vi "CRYGet Loose Curve array.vi"(8 "Unit Info In":T6={"Y unit In"="dB", "dB ref In"=1.0, "Y unit Out"="dB", "dB ref Out"=1.0, "Y unit Curve"="dB", "dB ref Curve"=1.0, "Y data  Curve"=0, "Y data Time"=0}, 9 "Loose Particle Waveform":bool, 11 "Additive Info":T2) -> (0 "Value Display Array":T4(array[cluster]), 1 "Value Unit Info Out":T5(array[cluster]), 2 "WMF Display Array":T4(array[cluster]), 3 "WFM Unit Info Out":T3[](array[typedef]), 4 "Curve Info Array Out":T1, 5 "WFM Info Array Out":T1)   [LabVIEW 2013]
uses:
  Typedef Control/CRYUnit Info Cluster.ctl
  Typedef Control/CRYUnit Info Out Cluster.ctl
  Typedef Control/CRYAnalysis CurveName Cluster.ctl
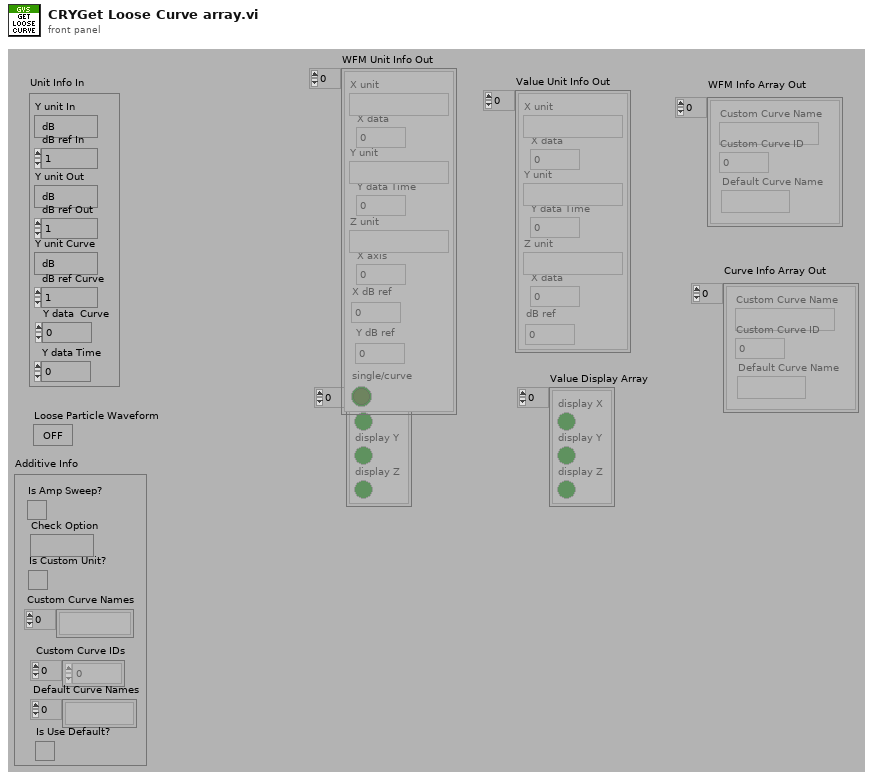
[diagram p1: front panel]
types:
  T1 = typedef "CRYAnalysis CurveName Cluster.ctl" = cluster{"Custom Curve Name":string, "Custom Curve ID":i32, "Default Curve Name":string}[]
  T2 = cluster{"Is Amp Sweep?":bool, "Check Option":string, "Is Custom Unit?":bool, "Custom Curve Names":string[], "Custom Curve IDs":i32[], "Default Curve Names":string[], "Is Use Default?":bool}
  T3 = typedef "CRYUnit Info Out Cluster.ctl" = cluster{"X unit":string, "X data":u16, "Y unit":string, "Y data Time":u16, "Z unit":string, "X axis":u16, "X dB ref":dbl, "Y dB ref":dbl, "single/curve":bool}
  T4 = cluster{"display X":bool, "display Y":bool, "display Z":bool}[]
  T5 = cluster{"X unit":string, "X data":u16, "Y unit":string, "Y data Time":u16, "Z unit":string, "X data":u16, "dB ref":dbl}[]
  T6 = typedef "CRYUnit Info Cluster.ctl" = cluster{"Y unit In":string, "dB ref In":dbl, "Y unit Out":string, "dB ref Out":dbl, "Y unit Curve":string, "dB ref Curve":dbl, "Y data  Curve":u16, "Y data Time":u16}
  T7 = cluster{"display X":bool, "display Y":bool, "display Z":bool}
  T8 = enum32{"English", "Chinese", "Korean", "Japanese", "Russian", "Chinese traditional"}
  T9 = cluster{"X unit":string, "X data":u16, "Y unit Curve":string, "Y data  Curve":u16, "Z unit":string, "X data":u16, "dB ref Curve":dbl, "dB ref Curve":dbl, "display X":bool}
  T10 = cluster{"X unit":string, "X data":u16, "Y unit Curve":string, "Y data  Curve":u16, "Z unit":string, "X data":u16, "dB ref Curve":dbl, "dB ref Curve":dbl, "display X":bool}[]
  T11 = cluster{"X unit":string, "X data":u16, "Y unit":string, "X data":u16, "Z unit":string, "X data":u16, "dB ref In":dbl}
  T12 = cluster{"X unit":string, "X data":u16, "Y unit":string, "X data":u16, "Z unit":string, "X data":u16, "dB ref In":dbl}[]
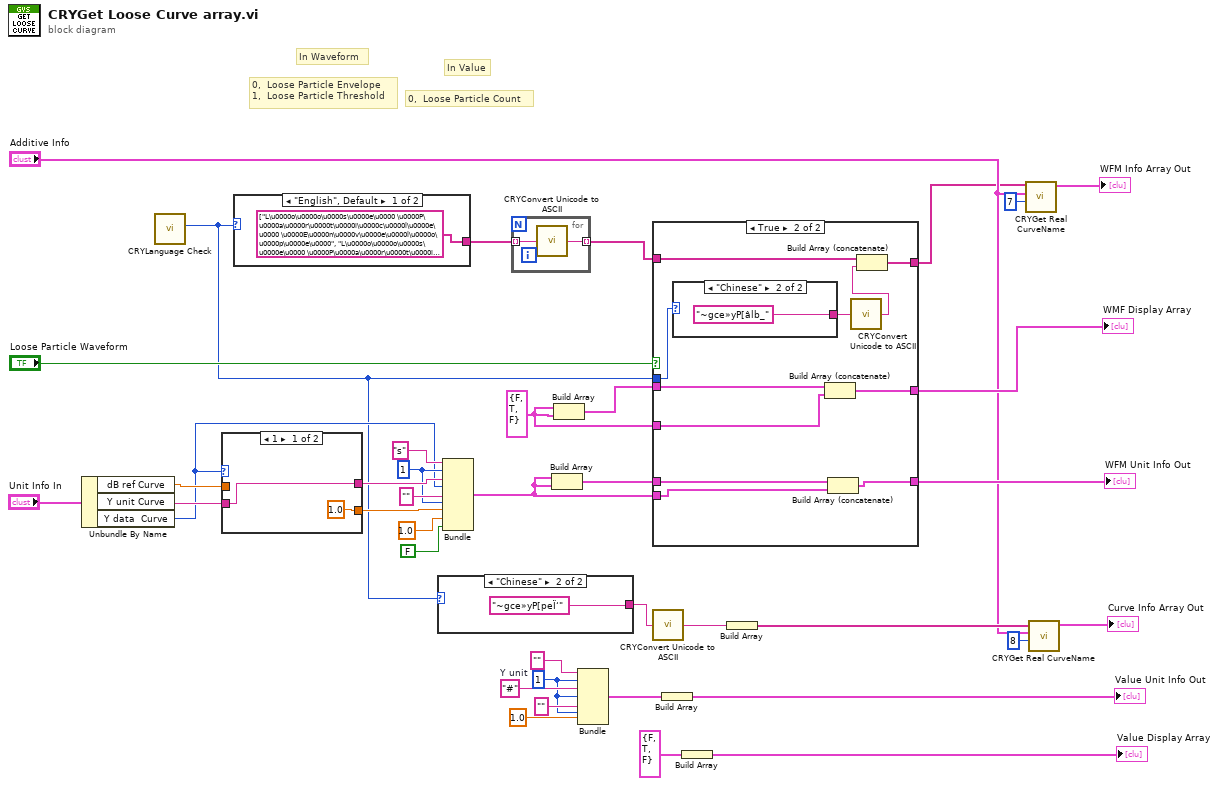
[diagram p0: block diagram]
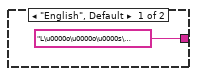
[diagram p2: hidden frame]
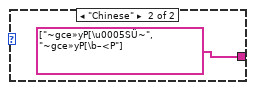
[diagram p3: hidden frame]
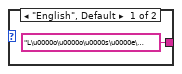
[diagram p5: hidden frame]
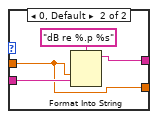
[diagram p6: hidden frame]
diagram:
  w25 = "#"  # Y unit
  w24 = u16 1 ("X data")
  w16 = T7 {"display X"=FALSE, "display Y"=TRUE, "display Z"=FALSE}
  w33 = u16 1 ("X data")
  # "In Waveform"
  # "In Value"
  # "0,  Loose Particle Count"
  # "0,  Loose Particle Envelope\n1,  Loose Particle Threshold"
  n1 = Unbundle By Name("Unit Info In") -> ("dB ref Curve"=w32:dbl, "Y unit Curve"=w31:string, "Y data  Curve"=w22:u16)
  n2 = call "CRYLanguage Check.vi"() -> ("Language"=w2:T8)  [unwired: 10 in, 1 out]
  n3 = case shown="1" w22 {
    tunnel: [w41 w43] -> w34
    tunnel: w32 -> [_ w42]
    tunnel: w31 -> [w41 w44]
    tunnel: [1.0 ("dB ref In") w42] -> w30
    frame 1 {
    }
    frame 0, Default {
      n4 = Format Into String(format string="dB re %.p %s", w42, w44) -> (resulting string=w43:string)  [unwired: 2 in, 1 out]
    }
  }
  n5 = case shown="\"English\", Default" w2 {
    tunnel: [string[] ["L\u0000o\u0000o\u0000s\u0000e\u0000 \u0000P\u0000a\u0000r\u0000t\u0000i\u0000c\u0000l\u0000e\u0000 \u0000E\u0000n\u0000v\u0000e\u0000l\u0000o\u0000p\u0000e\u0000", "L\u0000o\u0000o\u0000s\u0000e\u0000 \u0000P\u0000a\u0000r\u0000t\u0000i\u0000c\u0000l\u0000e\u0000 \u0000T\u0000h\u0000r\u0000e\u0000s\u0000h\u0000o\u0000l\u0000d\u0000"] string[] ["~gce»yP[\u0005SÜ~", "~gce»yP[\b–<P"]] -> w5
    frame "English", Default {
    }
    frame "Chinese" {
    }
  }
  n6 = case shown="\"Chinese\"" w2 {
    tunnel: ["L\u0000o\u0000o\u0000s\u0000e\u0000 \u0000P\u0000a\u0000r\u0000t\u0000i\u0000c\u0000l\u0000e\u0000 \u0000C\u0000o\u0000u\u0000n\u0000t\u0000" ("String 2") "~gce»yP[peÏ‘" ("Unicode")] -> w4
    frame "English", Default {
    }
    frame "Chinese" {
    }
  }
  n7 = Bundle("X unit"="s", "X data"=w33, "Y unit Curve"=w34, "Y data  Curve"=w22, "Z unit"="", "X data"=w33, "dB ref Curve"=w30, "dB ref Curve"=1.0, "display X"=FALSE) -> (w15:T9)  [unwired: 1 in]
  n8 = for {
    tunnel: [w51] -> w6 mode=indexing
    tunnel: w5 -> [w50] mode=indexing
    n9 = call "CRYConvert Unicode to ASCII.vi"("Unicode"=w50) -> ("ASCII"=w51:string)  [unwired: 4 in]
  }
  n10 = Build Array(w15, w15) -> (w19:T10)
  n11 = Build Array(w16, w16) -> (w20:T4)
  n12 = Bundle("X unit"="", "X data"=w24, "Y unit"=w25, "X data"=w24, "Z unit"="", "X data"=w24, "dB ref In"=1.0) -> (w26:T11)  [unwired: 1 in]
  n13 = case shown="True" "Loose Particle Waveform" {
    tunnel: w6 -> [w54 w65]
    tunnel: [w54 w64] -> w10
    tunnel: w20 -> [w53 w63]
    tunnel: w19 -> [w52 w60]
    tunnel: [w53 w61] -> w18
    tunnel: [w52 w59] -> w17
    tunnel: w16 -> [_ w62]
    tunnel: w15 -> [_ w58]
    tunnel: w2 -> [_ w57]
    frame False {
    }
    frame True {
      n14 = case shown="\"Chinese\"" w57 {
        tunnel: ["L\u0000o\u0000o\u0000s\u0000e\u0000 \u0000P\u0000a\u0000r\u0000t\u0000i\u0000c\u0000l\u0000e\u0000 \u0000W\u0000a\u0000v\u0000e\u0000f\u0000o\u0000r\u0000m\u0000" ("String 2") "~gce»yP[âlb_" ("Unicode")] -> w56
        frame "English", Default {
        }
        frame "Chinese" {
        }
      }
      n15 = Build Array (concatenate)(w63, w62) -> (w61:T4)
      n16 = Build Array (concatenate)(w60, w58) -> (w59:T10)
      n17 = call "CRYConvert Unicode to ASCII.vi"("Unicode"=w56) -> ("ASCII"=w55:string)  [unwired: 4 in]
      n18 = Build Array (concatenate)(w65, w55) -> (w64:string[])
    }
  }
  "WMF Display Array" <- w18
  "WFM Unit Info Out" <- w17
  n19 = call "CRYConvert Unicode to ASCII.vi"("Unicode"=w4) -> ("ASCII"=w3:string)  [unwired: 4 in]
  n20 = Build Array(w26) -> (→"Value Unit Info Out":T12)
  n21 = Build Array(T7 {"display X"=FALSE, "display Y"=TRUE, "display Z"=FALSE}) -> (→"Value Display Array":T4)
  n22 = Build Array(w3) -> (w13:string[])
  n23 = call "CRYGet Real CurveName.vi"("Key No"=7, "Additive Info"="Additive Info", "CurveArrayByType"=w10) -> ("Curve Info Array Out"=→"WFM Info Array Out":T1)  [unwired: 8 in]
  n24 = call "CRYGet Real CurveName.vi"("Key No"=8, "Additive Info"="Additive Info", "CurveArrayByType"=w13) -> ("Curve Info Array Out"=→"Curve Info Array Out":T1)  [unwired: 8 in]
